vi "Ref plot window caller.vi"(8 "error in (no error)":errorcluster, 10 "Bring to front (F)":bool) -> (1 "Window is open":bool)   [LabVIEW 2020]
uses:
  Global Variables/General Globals.vi
panel:
  # "Calls the \"Ref Plots Window\" window dynamically."
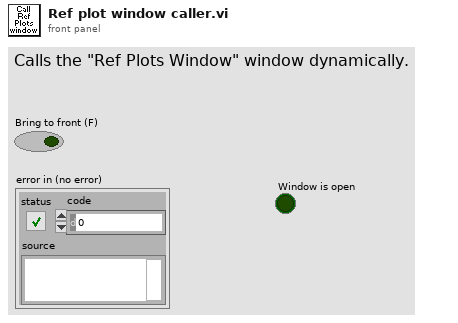
[diagram p1: front panel]
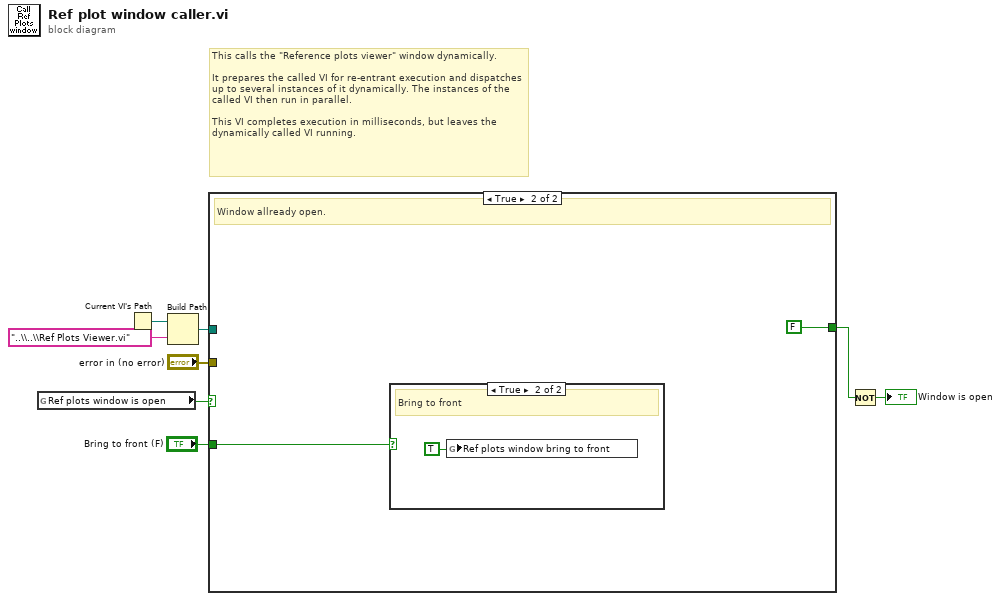
[diagram p0: block diagram]
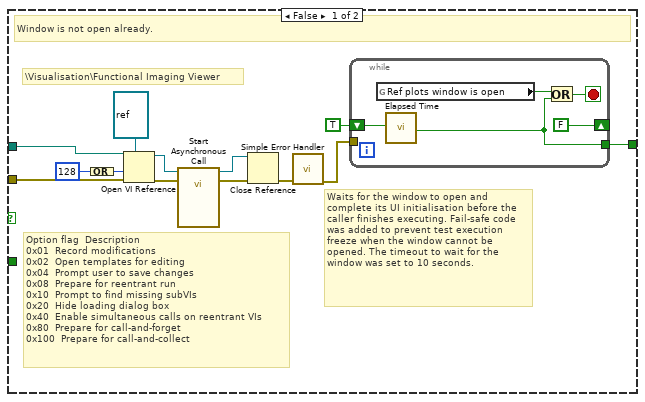
[diagram p2: hidden frame]
diagram:
  # "This calls the \"Reference plots viewer\" window dynamically.\n\nIt prepares the called VI for re-entrant execution and dispatches up to several instances of it dynamically. The instances of the called VI then run in parallel.\n\nThis VI completes execution in milliseconds, but leaves the dynamically called VI running."
  n1 = global read "General Globals.vi" "Ref plots window is open"() -> (w4:bool)
  n2 = Current VI's Path() -> (path=w7:path)
  n3 = Build Path(base path=w7, name or relative path="..\\..\\Ref Plots Viewer.vi") -> (appended path=w6:path)
  n4 = case shown="True" w4 {
    tunnel: "error in (no error)" -> [w11 _]
    tunnel: w6 -> [w10 _]
    tunnel: [w9 FALSE ("Time has Elapsed")] -> w2
    tunnel: "Bring to front (F)" -> [_ w27]
    frame False {
      # "\\Visualisation\\Functional Imaging Viewer"
      # "Waits for the window to open and complete its UI initialisation before the caller finishes executing. Fail-safe code was added to prevent test execution freeze when the window cannot be opened. The timeout to wait for the window was set to 10 seconds."
      # "Option flag \tDescription\n0x01 \tRecord modifications\n0x02 \tOpen templates for editing\n0x04 \tPrompt user to save changes\n0x08 \tPrepare for reentrant run\n0x10 \tPrompt to find missing subVIs\n0x20 \tHide loading dialog box\n0x40 \tEnable simultaneous calls on reentrant VIs\n0x80 \tPrepare for call-and-forget\n0x100 \tPrepare for call-and-collect"
      # "Window is not open already."
      n5 = Compound Arithmetic op=OR(128) -> (w15:i32)
      n6 = Open VI Reference(type specifier VI Refnum (for type only)=refnum<vi> refnum, vi path=w10, options=w15, error in (no error)=w11) -> (vi reference=w14:refnum<vi>, error out=w13:errorcluster)  [unwired: 2 in]
      n7 = call-by-ref "Start Asynchronous Call"(reference=w14, error in=w13) -> (reference out=w20:refnum<vi>, error out=w19:errorcluster)  [unwired: 12 in]
      n8 = Close Reference(reference=w20, error in (no error)=w19) -> (error out=w21:errorcluster)
      n9 = call <vilib>:"Simple Error Handler.vi"("error in (no error)"=w21) -> ("error out"=w17:errorcluster)  [unwired: 4 in, 4 out]
      n10 = while {
        shift-right: [FALSE ("Reset")] -> _
        shift-left: TRUE ("Reset") -> [w25]
        tunnel: w17 -> [_]
        tunnel: [w23] -> w9
        stop <- w26 stop-if-true
        n11 = global read "General Globals.vi" "Ref plots window is open"() -> (w22:bool)
        n12 = call "Elapsed Time"("Reset"=w25) -> ("Time has Elapsed"=w23:bool)  [unwired: 11 in, 7 out]
        n13 = Or(x=w22, y=w23) -> (x .or. y?=w26:bool)
      }
    }
    frame True {
      # "Window allready open."
      n14 = case shown="True" w27 {
        frame False {
        }
        frame True {
          # "Bring to front"
          n15 = global write "General Globals.vi" "Ref plots window bring to front"(TRUE ("\"Values Check\" report window is open")) -> ()
        }
      }
    }
  }
  n16 = Not(x=w2) -> (.not. x?=→"Window is open":bool)
